vi "Get IP Address.vi"() -> ()   [LabVIEW 2013]
panel:
  out "error out":errorcluster
  in  "error in (no error)":errorcluster
  out "LAN Setting":T1
  # "Get IP Address"
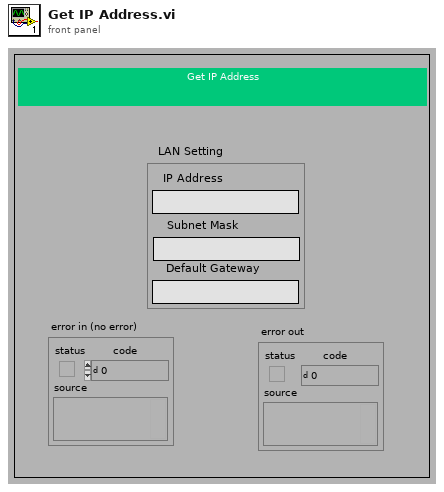
[diagram p1: front panel]
types:
  T1 = cluster{"IP Address":string, "Subnet Mask":string, "Default Gateway":string}
  T2 = cluster{"[0]":string, "[1]":string, "[2]":string}
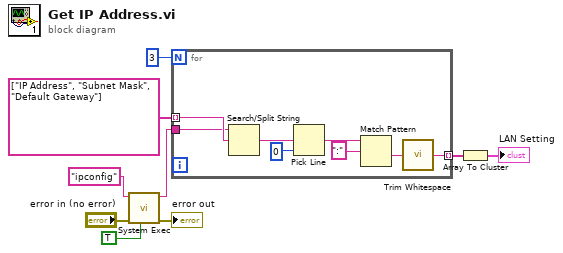
[diagram p0: block diagram]
diagram:
  n1 = call <vilib>:"System Exec.vi"("run minimized? (F)"=TRUE, "error in (no error)"="error in (no error)", "command line"="ipconfig") -> ("error out"=→"error out":errorcluster, "standard output"=w6:string)  [unwired: 5 in, 2 out]
  n2 = for {
    N: 3 -> [_]
    tunnel: string[] ["IP Address", "Subnet Mask", "Default Gateway"] -> [w17] mode=indexing
    tunnel: [w11] -> w4 mode=indexing
    tunnel: w6 -> [w10]
    n3 = Search/Split String(string=w10, search string/char (-)=w17) -> (match + rest of string=w15:string)  [unwired: 1 in, 2 out]
    n4 = Pick Line(multi-line string=w15, line index=0) -> (output string=w13:string)  [unwired: 1 in]
    n5 = Match Pattern(string=w13, regular expression=":") -> (after substring=w12:string)  [unwired: 1 in, 3 out]
    n6 = call <vilib>:"Trim Whitespace.vi"("string"=w12) -> ("trimmed string"=w11:string)  [unwired: 1 in]
  }
  n7 = Array To Cluster(array=w4) -> (cluster=→"LAN Setting":T2)
